vi "Cull and Group Peg.vi"(6 "Line Border":cluster{"Top":dbl, "Bottom":dbl}={"Top"=6.0, "Bottom"=1.0}, 9 "Score Cutoff":dbl=50.0, 10 "Sorted Data":dbl[][](array[numeric])) -> (0 "Rect Out":T3 {"Bottom" format="%#_3g"; "Right" format="%#_3g"; "Top" format="%#_3g"; "Left" format="%#_3g"}, 1 "Line Out":T1, 2 "Top Score Out":dbl, 3 "Center Out":T2)   [LabVIEW 2017, in "VisionSystem.lvlib"]
doc: "Examine the particle measurements to find the most likely pair that make up the target. This mostly compares the edges of the bounding boxes. It then returns information about the overall target, notably the rectangle sourrounding the particles, the vertical line that bisects the target, and the center of the top particle."
uses:
  VisionSystem.lvlib
  Cluster_UI DBL Box.ctl
  Cluster_DBL Point.ctl
  Cluster_Line.ctl
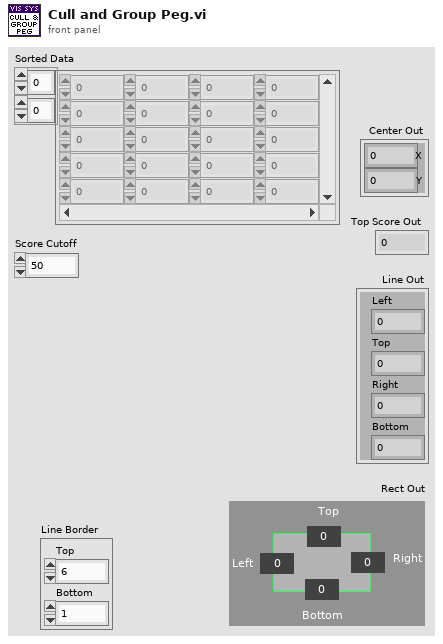
[diagram p1: front panel]
types:
  T1 = typedef "VisionSystem.lvlib/Cluster_Line.ctl" = cluster{"Left":dbl, "Top":dbl, "Right":dbl, "Bottom":dbl}
  T2 = typedef "VisionSystem.lvlib/Cluster_DBL Point.ctl" = cluster{"X":dbl, "Y":dbl}
  T3 = typedef "VisionSystem.lvlib/Cluster_UI DBL Box.ctl" = cluster{"Left":dbl, "Top":dbl, "Right":dbl, "Bottom":dbl}
  T4 = typedef "Particle Parameters" = i32
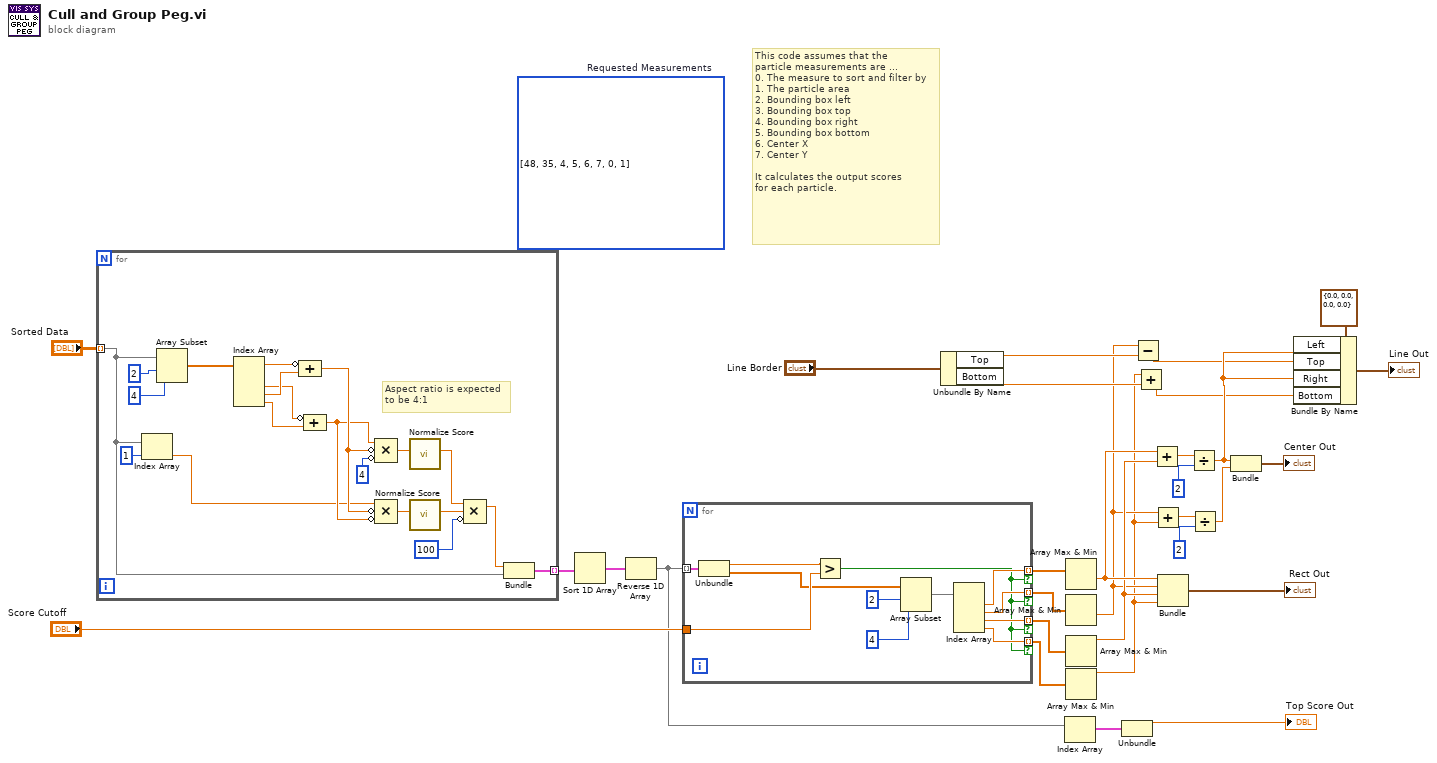
[diagram p0: block diagram]
diagram:
  (unwired) T4[] [48, 35, 4, 5, 6, 7, 0, 1] items=["Center of Mass X", "Center of Mass Y", "First Pixel X", "First Pixel Y", "Bounding Rect Left", "Bounding Rect Top", "Bounding Rect Right", "Bounding Rect Bottom", "Max Feret Diameter Start X", "Max Feret Diameter Start Y", "Max Feret Diameter End X", "Max Feret Diameter End Y", "Max Horiz. Segment Length Left", "Max Horiz. Segment Length Right", "Max Horiz. Segment Length Row", "-", "Bounding Rect Width", "Bounding Rect Height", "Bounding Rect Diagonal", "Perimeter", "Convex Hull Perimeter", "Holes' Perimeter", "Max Feret Diameter", "Equivalent Ellipse Major Axis", "Equivalent Ellipse Minor Axis", "Equivalent Ellipse Minor Axis (Feret)", "Equivalent Rect Long Side", "Equivalent Rect Short Side", "Equivalent Rect Diagonal", "Equivalent Rect Short Side (Feret)", "Average Horiz. Segment Length", "Average Vert. Segment Length", "Hydraulic Radius", "Waddel Disk Diameter", "-", "Area", "Holes' Area", "Particle & Holes' Area", "Convex Hull Area", "Image Area", "-", "Number of Holes", "Number of Horiz. Segments", "Number of Vert. Segments", "-", "Orientation", "Max Feret Diameter Orientation", "-", "% Area/Image Area", "% Area/(Particle & Holes' Area)", "Ratio of Equivalent Ellipse Axes", "Ratio of Equivalent Rect Sides", "-", "Elongation Factor", "Compactness Factor", "Heywood Circularity Factor", "Type Factor", "-", "Sum X", "Sum Y", "Sum XX", "Sum XY", "Sum YY", "Sum XXX", "Sum XXY", "Sum XYY", "Sum YYY", "-", "Moment of Inertia XX", "Moment of Inertia XY", "Moment of Inertia YY", "Moment of Inertia XXX", "Moment of Inertia XXY", "Moment of Inertia XYY", "Moment of Inertia YYY", "Norm. Moment of Inertia XX", "Norm. Moment of Inertia XY", "Norm. Moment of Inertia YY", "Norm. Moment of Inertia XXX", "Norm. Moment of Inertia XXY", "Norm. Moment of Inertia XYY", "Norm. Moment of Inertia YYY", "Hu Moment 1", "Hu Moment 2", "Hu Moment 3", "Hu Moment 4", "Hu Moment 5", "Hu Moment 6", "Hu Moment 7"]  # Requested Measurements
  # "This code assumes that the\nparticle measurements are ...\n0. The measure to sort and filter by\n1. The particle area\n2. Bounding box left\n3. Bounding box top\n4. Bounding box right\n5. Bounding box bottom\n6. Center X\n7. Center Y\n\nIt calculates the output scores\nfor each particle."
  n1 = for {
    tunnel: "Sorted Data" -> [w35] mode=indexing
    tunnel: [w33] -> w29 mode=indexing
    # "Aspect ratio is expected\nto be 4:1"
    n2 = Index Array(array=w35, index=1) -> (element=w31:dbl)
    n3 = Array Subset(array=w35, index=2, length=4) -> (w48:dbl[])
    n4 = Index Array(array=w48) -> (element #1=w46:dbl, element #2=w44:dbl, element #3=w47:dbl, element #4=w45:dbl)  [unwired: 4 in]
    n5 = Compound Arithmetic op=ADD(invert w46, w47) -> (w41:dbl)
    n6 = Compound Arithmetic op=ADD(invert w44, w45) -> (w40:dbl)
    n7 = Compound Arithmetic op=MULTIPLY(w40, invert w41, invert 4 ("length")) -> (w42:dbl)
    n8 = Compound Arithmetic op=MULTIPLY(w31, invert w41, invert w40) -> (w39:dbl)
    n9 = call "Normalize Score.vi"("Value"=w42) -> ("Score"=w38:dbl)  [unwired: 10 in]
    n10 = call "Normalize Score.vi"("Value"=w39) -> ("Score"=w37:dbl)  [unwired: 10 in]
    n11 = Compound Arithmetic op=MULTIPLY(w38, w37, invert 100 ("length")) -> (w34:dbl)
    n12 = Bundle(w34, "Sorted Data"=w35) -> (w33:cluster{dbl, "Sorted Data":dbl[]})  [unwired: 1 in]
  }
  n13 = Sort 1D Array(array=w29) -> (sorted array=w22:cluster{dbl, "Sorted Data":dbl[]}[])
  n14 = Reverse 1D Array(array=w22) -> (reversed array=w19:cluster{dbl, "Sorted Data":dbl[]}[])
  n15 = for {
    tunnel: w19 -> [w62] mode=indexing
    tunnel: "Score Cutoff" -> [w60]
    tunnel: [w55] -> w27 mode=indexing if=w51
    tunnel: [w54] -> w26 mode=indexing if=w51
    tunnel: [w53] -> w25 mode=indexing if=w51
    tunnel: [w52] -> w24 mode=indexing if=w51
    n16 = Unbundle(w62) -> (w61:dbl, "Sorted Data"=w56:dbl[])
    n17 = Greater?(x=w61, y=w60) -> (0:w51:bool)
    n18 = Array Subset(array=w56, index=2, length=4) -> (w59:dbl[])
    n19 = Index Array(array=w59) -> (element #1=w55:dbl, element #2=w54:dbl, element #3=w53:dbl, element #4=w52:dbl)  [unwired: 4 in]
  }
  n20 = Unbundle By Name("Line Border") -> ("Top"=w5:dbl, "Bottom"=w6:dbl)
  n21 = Index Array(array=w19) -> (element=w21:cluster{dbl, "Sorted Data":dbl[]})  [unwired: 1 in]
  n22 = Array Max & Min(array=w27) -> (min value=w9:dbl)  [unwired: 3 out]
  n23 = Array Max & Min(array=w26) -> (min value=w4:dbl)  [unwired: 3 out]
  n24 = Array Max & Min(array=w25) -> (max value=w8:dbl)  [unwired: 3 out]
  n25 = Array Max & Min(array=w24) -> (max value=w3:dbl)  [unwired: 3 out]
  n26 = Unbundle(w21) -> (→"Top Score Out":dbl)  [unwired: 1 out]
  n27 = Subtract(x=w4, y=w5) -> (x-y=w1:dbl)
  n28 = Add(x=w3, y=w6) -> (x+y=w2:dbl)
  n29 = Add(x=w9, y=w8) -> (x+y=w17:dbl)
  n30 = Add(x=w4, y=w3) -> (x+y=w16:dbl)
  n31 = Bundle(w9, w4, w8, w3) -> (→"Rect Out":cluster{dbl, dbl, dbl, dbl})  [unwired: 1 in]
  n32 = Divide(x=w17, y=2 ("index")) -> (x/y=w7:dbl)
  n33 = Divide(x=w16, y=2 ("index")) -> (x/y=w14:dbl)
  n34 = Bundle(w7, w14) -> (→"Center Out":cluster{dbl, dbl})  [unwired: 1 in]
  n35 = Bundle By Name(cluster=T1 {"Left"=0.0, "Top"=0.0, "Right"=0.0, "Bottom"=0.0} ("Line Out"), "Left"=w7, "Top"=w1, "Right"=w7, "Bottom"=w2) -> (→"Line Out":T1)
